vi "Configure Volume Flow.vi"(8 "error in (no error)":errorcluster, 9 "Temperature (20)":dbl=20.0, 10 "Pressure (101.325 kPaa)":dbl=101.325, 11 "VISA resource name":refnum<visa-resource-name>) -> (0 "error out":errorcluster, 3 "VISA resource name out":refnum<visa-resource-name>)   [LabVIEW 2023, in "Fluke Molbox 1 Plus.lvlib"]
doc: "Configures the pressure and temerpature conditions that are used to calculate the volume flow unit of measurement. The flow volume units \"ccm\", \"lm\", \"lh\", \"m3m\", \"m3h\", \"cfm\", and \"cfh\" require pressure and a temperature conditions to be specified by the user."
uses:
  Fluke Molbox 1 Plus.lvlib
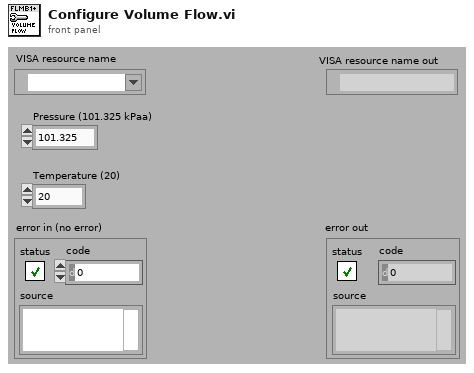
[diagram p1: front panel]
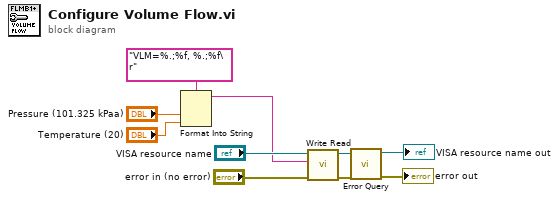
[diagram p0: block diagram]
diagram:
  n1 = Format Into String(format string="VLM=%.;%f, %.;%f\r", "Pressure (101.325 kPaa)", "Temperature (20)") -> (resulting string=w5:string)  [unwired: 2 in, 1 out]
  n2 = call "Write Read.vi"("error in (no error)"="error in (no error)", "Write String"=w5, "VISA resource name"="VISA resource name") -> ("error out"=w3:errorcluster, "VISA resource name out"=w4:refnum<visa-resource-name>)  [unwired: 6 in, 1 out]
  n3 = call "Error Query.vi"("error in (no error)"=w3, "VISA resource name"=w4) -> ("error out"=→"error out":errorcluster, "VISA resource name out"=→"VISA resource name out":refnum<visa-resource-name>)  [unwired: 6 in, 2 out]
